vi "Set TDMS Channel Property.vi"(5 "Property Value":variant, 7 "Property Name":string, 8 "error in (no error)":errorcluster, 9 "Channel Name in":string, 10 "Group Name in":string, 11 "TDMS Log File in":refnum<class "TDMS Log File.lvclass">) -> (0 "error out":errorcluster, 1 "Channel Name out":string, 2 "Group Name out":string, 3 "TDMS Log File out":refnum<class "TDMS Log File.lvclass">)   [LabVIEW 2015, in "TDMS Log File.lvclass"]
uses:
  TDMS Log File.lvclass
  TDMS Log File.lvclass/TDMS Log File.ctl
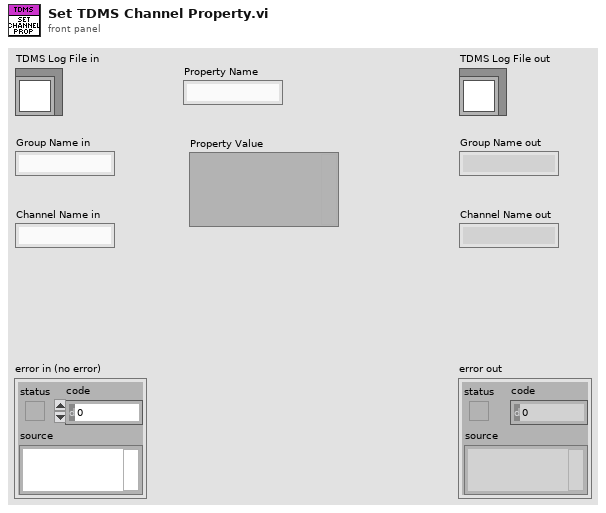
[diagram p1: front panel]
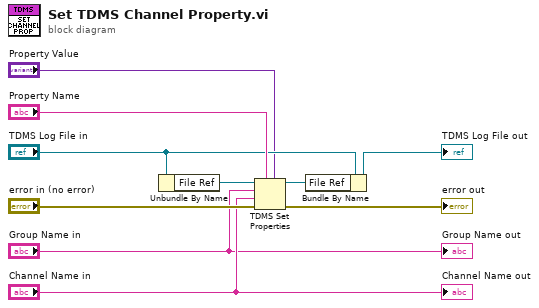
[diagram p0: block diagram]
diagram:
  n1 = Unbundle By Name("TDMS Log File in") -> ("File Ref"=w4:refnum<k34>)
  n2 = TDMS Set Properties(5:"Property Value", 7:"Property Name", 8:"error in (no error)", 9:"Channel Name in", 10:"Group Name in", 11:w4) -> (0:→"error out":errorcluster, 3:w3:refnum<k34>)  [unwired: 2 out]
  n3 = Bundle By Name(cluster="TDMS Log File in", "File Ref"=w3) -> (→"TDMS Log File out":refnum<class "TDMS Log File.lvclass">)
  "Group Name out" <- "Group Name in"
  "Channel Name out" <- "Channel Name in"
